vi "Pulse Timer.vi"(8 "error in":errorcluster, 9 "preset time (ms)":i32=1000, 11 "input":bool) -> (0 "error out":errorcluster, 1 "elapsed time (ms)":i32, 3 "output":bool)   [LabVIEW 2012, in "毫秒定时器.lvlib"]
uses:
  <vilib>/ptbypt/NI_PtbyPt.lvlib
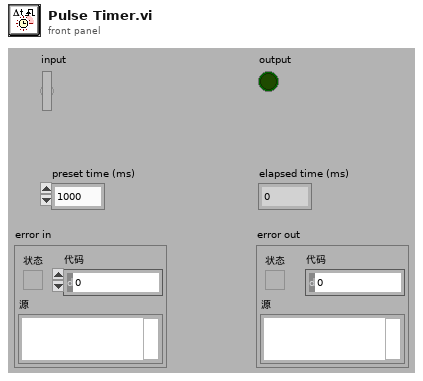
[diagram p1: front panel]
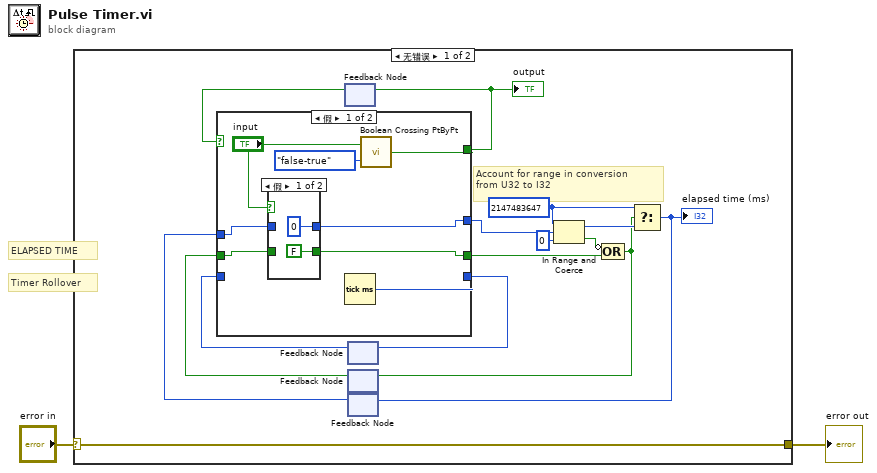
[diagram p0: block diagram]
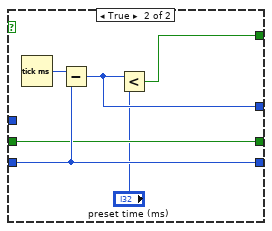
[diagram p3: hidden frame]
diagram:
  # "ELAPSED TIME"
  # "Timer Rollover"
  n1 = case shown="无错误" "error in" {
    selector: "error in" -> [w17 w36]
    tunnel: [w17 w36] -> w1
    frame No Error {
      w11 = u32 2147483647 ("upper limit")
      # "Account for range in conversion\nfrom U32 to I32"
      n2 = feedback #1() -> (w13:bool)  [unwired: 1 in]
      n3 = feedback #2() -> (w15:u32)  [unwired: 1 in]
      n4 = feedback #3() -> (w4:bool)  [unwired: 1 in]
      n5 = feedback #4() -> (w12:u32)  [unwired: 1 in]
      n6 = case shown="假" w13 {
        tunnel: [w24 w33] -> w14
        tunnel: [w22 w32] -> w7
        tunnel: [w23 w34] -> w16
        tunnel: w15 -> [_ w34]
        tunnel: w12 -> [w20 _]
        tunnel: w4 -> [w18 w31]
        tunnel: [w19 w31] -> w3
        frame False {
          n7 = case shown="假" "input" {
            tunnel: [0 ("ELAPSED TIME (ms)") w29] -> w22
            tunnel: w20 -> [_ w29]
            tunnel: [FALSE w28] -> w19
            tunnel: w18 -> [_ w28]
            frame False {
            }
            frame True {
            }
          }
          n8 = Tick Count (ms)() -> (millisecond timer value=w23:u32)
          n9 = call <vilib>:"Boolean Crossing PtByPt.vi"("direction"=enum16{"either", "false-true", "true-false"}."false-true", "input"="input") -> ("crossing"=w24:bool)  [unwired: 1 in]
        }
        frame True {
          n10 = Tick Count (ms)() -> (millisecond timer value=w35:u32)
          n11 = Subtract(x=w35, y=w34) -> (x-y=w32:u32)
          n12 = Less?(x=w32, y="preset time (ms)") -> (x < y?=w33:bool)
        }
      }
      "output" <- w14
      n13 = feedback-in #1(w14) -> ()
      n14 = feedback-in #2(w16) -> ()
      n15 = In Range and Coerce(upper limit=w11, x=w7, lower limit=u32 0) -> (coerced(x)=w10:u32, In Range?=w9:bool)
      n16 = Compound Arithmetic op=OR(invert w9, w3) -> (w5:bool)
      n17 = feedback-in #3(w5) -> ()
      n18 = Select(t=w11, s=w5, f=w10) -> (s? t:f=w6:u32)
      "elapsed time (ms)" <- w6
      n19 = feedback-in #4(w6) -> ()
    }
    frame Error {
    }
  }
  "error out" <- w1
